vi "Fields Update PI Steps.vi"(8 "error in (no error)":errorcluster, 11 "Connection Refnum":T1) -> (0 "error out":errorcluster, 3 "dup Connection Refnum":T1)   [LabVIEW 2011]
uses:
  SI.LIB/ODBC/SQL Controls/Connection Refnum.ctl
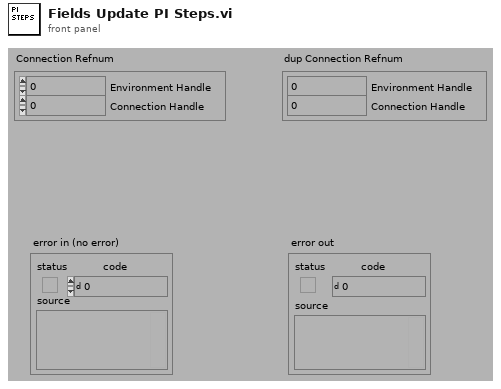
[diagram p1: front panel]
types:
  T1 = typedef "Connection Refnum.ctl" = cluster{"Environment Handle":i32, "Connection Handle":i32}
  T2 = typedef "Field Record.ctl" = cluster{"ixField":i32, "iSequenceOrder":i32, "sxFieldId":string, "sxSequenceId":string, "sDisplayName":string, "sValue":string, "sUnits":string, "nDataType":T3, "nNextItem":T4, "fSystem":bool, "fSystemValue":bool, "fRequired":bool, "fSetAtTest":bool, "fTestField":bool, "fDeleted":bool, "fIndexed":bool, "fFreeList":bool}
  T3 = typedef "Field DataTypes.ctl" = enum32{"text", "numeric", "list", "timestamp", "boolean"}
  T4 = typedef "Field NextItem.ctl" = enum32{"Reset", "Retain", "Auto-Increment"}
  T5 = typedef "Step Record.ctl" = cluster{"ixStep":i32, "sxSequenceId":string, "sxTestId":string, "iIndex":i32, "iRepeat":i32, "iQuickMode":i32, "sTag":string, "sDatasheetsCSV":string, "bConfiguration":string}
  T6 = typedef "PI Test Parameters.ctl" = cluster{"Measurement":T7, "Limit":T8}
  T7 = typedef "PI Measurement Cluster.ctl" = cluster{"sxFieldId":string, "sValue":string, "nDataType":enum16{"Scalar", "Enumeration"}, "sUnits":string, "sDisplayName":string}
  T8 = typedef "PI Limit Parameters.ctl" = cluster{"Limits On":bool, "Limits":T9[]}
  T9 = typedef "PI Limit Definition.ctl" = cluster{"nComparison":T10, "sValue":string}
  T10 = typedef "PI Limit Comparison.ctl" = enum16{">", ">=", "<", "<=", "<>", "="}
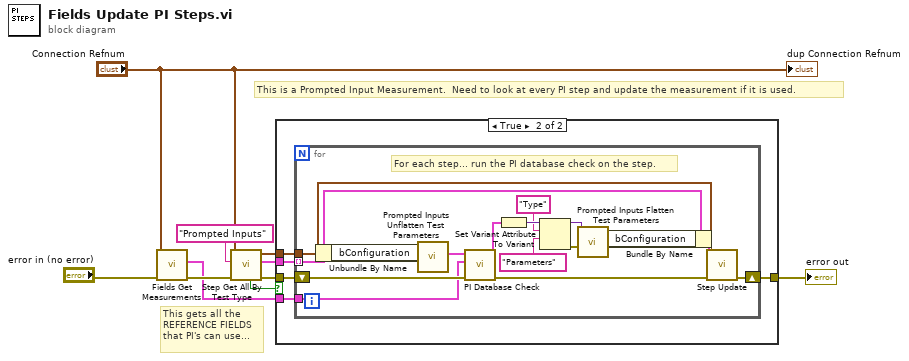
[diagram p0: block diagram]
diagram:
  # "This gets all the\nREFERENCE FIELDS\nthat PI's can use..."
  # "This is a Prompted Input Measurement.  Need to look at every PI step and update the measurement if it is used."
  n1 = call "Fields Get Measurements.vi"("error in (no error)"="error in (no error)", "Connection Refnum"="Connection Refnum") -> ("error out"=w10:errorcluster, "Measurement Fields"=w4:T2[])  [unwired: 1 in, 7 out]
  n2 = call "Step Get All By Test Type.vi"("error in (no error)"=w10, "sxTestId (\"\")"="Prompted Inputs" ("Test Type"), "Connection Refnum"="Connection Refnum") -> ("error out"=w7:errorcluster, "Sequence Steps"=w5:T5[], "Connection Refnum"=w6:T1, "Data Present"=w8:bool)  [unwired: 1 in, 4 out]
  n3 = case shown="True" w8 {
    tunnel: [w11 w15] -> w2
    tunnel: w7 -> [w11 w16]
    tunnel: w6 -> [_ w12]
    tunnel: w5 -> [_ w14]
    tunnel: w4 -> [_ w13]
    frame False {
    }
    frame True {
      n4 = for {
        shift-right: [w20] -> w15
        shift-left: w16 -> [w32]
        tunnel: w14 -> [w23] mode=indexing
        tunnel: w13 -> [w18]
        tunnel: w12 -> [w17]
        # "For each step... run the PI database check on the step."
        n5 = Unbundle By Name(w23) -> ("bConfiguration"=w31:string)
        n6 = call "Prompted Inputs Unflatten Test Parameters.vi"("Parameter String"=w31) -> ("Prompted Inputs Test Parameters"=w30:T6)  [unwired: 1 in, 9 out]
        n7 = call "PI Database Check.vi"("error in (no error)"=w32, "PI Fields"=w18, "PI Test Parameters In"=w30) -> ("error out"=w21:errorcluster, "PI Test Parameters Out"=w24:T6)  [unwired: 7 out]
        n8 = To Variant(anything=w24) -> (Variant=w29:variant)
        n9 = Set Variant Attribute(Variant=w29, name="Type", value="Parameters" ("name")) -> (Variant out=w25:variant, error out=w28:errorcluster)  [unwired: 1 in, 1 out]
        n10 = call "Prompted Inputs Flatten Test Parameters.vi"("error in (no error)"=w28, "Parameter Variant"=w25) -> ("Parameter String"=w22:string)  [unwired: 9 out]
        n11 = Bundle By Name(cluster=w23, "bConfiguration"=w22) -> (w19:T5)
        n12 = call "Step Update.vi"("error in (no error)"=w21, "Step Record (empty)"=w19, "Connection Refnum"=w17) -> ("error out"=w20:errorcluster)  [unwired: 8 out]
      }
    }
  }
  "error out" <- w2
  "dup Connection Refnum" <- "Connection Refnum"
